vi "Get Ideal Aperture Time.vi"(0 "Measured Power (dBm)":dbl format="%#_13g", 5 "Total Aperture Time Limit (s)":dbl=120.0 format="%#_13g", 9 "Maximum Two Sigma Uncertainty (dB)":dbl=0.05 format="%#_13g", 11 "error in (no error)":errorcluster) -> (4 "Ideal Total Aperture time (s)":dbl, 6 "Ideal Number of Averages":dbl format="%.2f", 15 "error out":errorcluster)   [LabVIEW 2023, in "NI-568x RF Power Meter.lvlib" / "SG 2250 Path Accessor.lvclass"]
uses:
  SG 2250 Path Accessor.lvclass
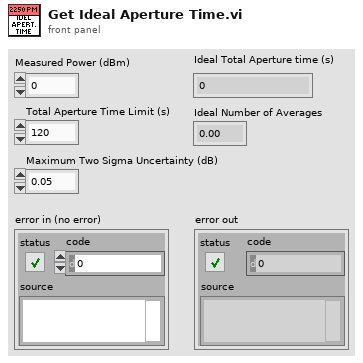
[diagram p1: front panel]
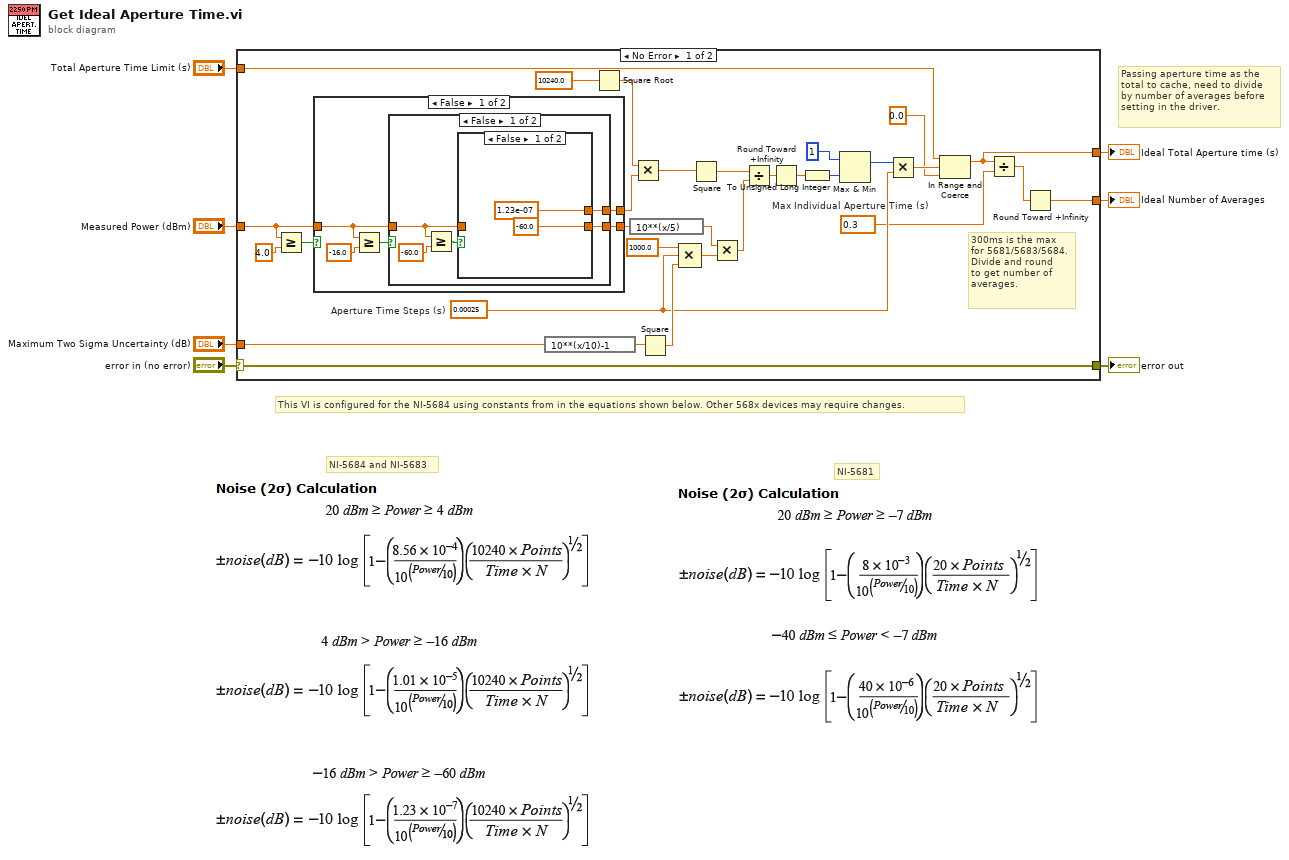
[diagram p0: block diagram]
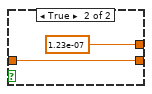
[diagram p2: hidden frame]
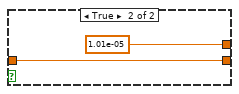
[diagram p3: hidden frame]
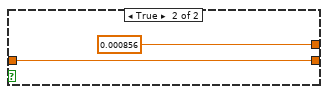
[diagram p4: hidden frame]
diagram:
  # "Passing aperture time as the\ntotal to cache, need to divide\nby number of averages before\nsetting in the driver."
  # "NI-5681"
  # "NI-5684 and NI-5683"
  # "This VI is configured for the NI-5684 using constants from in the equations shown below. Other 568x devices may require changes."
  n1 = case shown="No Error" "error in (no error)" {
    selector: "error in (no error)" -> [w16 w56]
    tunnel: "Measured Power (dBm)" -> [w32 _]
    tunnel: [w11 _] -> w6
    tunnel: [w16 w56] -> w4
    tunnel: [w13 _] -> w3
    tunnel: "Maximum Two Sigma Uncertainty (dB)" -> [w9 _]
    tunnel: "Total Aperture Time Limit (s)" -> [w8 _]
    frame No Error {
      w15 = 0.3  # Max Individual Aperture Time (s)
      w17 = 0.00025  # Aperture Time Steps (s)
      # "300ms is the max\nfor 5681/5683/5684.\nDivide and round\nto get number of\naverages."
      n2 = Greater Or Equal?(x=w32, y=4.0 ("upper limit")) -> (x >= y?=w34:bool)
      n3 = case shown="False" w34 {
        tunnel: w32 -> [w40 w55]
        tunnel: [w41 w55] -> w20
        tunnel: [w39 0.000856 ("t")] -> w33
        frame False {
          n4 = Greater Or Equal?(x=w40, y=-16.0 ("upper limit")) -> (x >= y?=w38:bool)
          n5 = case shown="False" w38 {
            tunnel: [w47 w52] -> w41
            tunnel: w40 -> [w44 w52]
            tunnel: [w46 1.01e-05 ("f")] -> w39
            frame False {
              n6 = Greater Or Equal?(x=w44, y=-60.0 ("upper limit")) -> (x >= y?=w43:bool)
              n7 = case shown="False" w43 {
                tunnel: [-60.0 ("Measured power (dBm)") w51] -> w47
                tunnel: [1.23e-07 ("f") 1.23e-07 ("f")] -> w46
                tunnel: w44 -> [_ w51]
                frame False {
                }
                frame True {
                }
              }
            }
            frame True {
            }
          }
        }
        frame True {
        }
      }
      n8 = expression code="10**(x/10)-1"(w9) -> (w26:dbl)
      n9 = Square Root(x=10240.0) -> (sqrt(x)=w35:dbl)
      n10 = expression code="10**(x/5)"(w20) -> (w29:dbl)
      n11 = Multiply(x=w35, y=w33) -> (x*y=w21:dbl)
      n12 = Square(x=w26) -> (x^2=w25:dbl)
      n13 = Compound Arithmetic op=MULTIPLY(1000.0 ("value"), w17, w25) -> (w19:dbl)
      n14 = Square(x=w21) -> (x^2=w27:dbl)
      n15 = Multiply(x=w29, y=w19) -> (x*y=w30:dbl)
      n16 = Divide(x=w27, y=w30) -> (x/y=w31:dbl)
      n17 = Round Toward +Infinity(x=w31) -> (ceil(x): smallest int >= x=w24:dbl)
      n18 = To Unsigned Long Integer(number=w24) -> (unsigned 32bit integer=w23:u32)
      n19 = Max & Min(x=u32 1, y=w23) -> (max(x,y)=w18:u32)  [unwired: 1 out]
      n20 = Multiply(x=w18, y=w17) -> (x*y=w12:dbl)
      n21 = In Range and Coerce(upper limit=w8, x=w12, lower limit=0.0) -> (coerced(x)=w11:dbl)  [unwired: 1 out]
      n22 = Divide(x=w11, y=w15) -> (x/y=w14:dbl)
      n23 = Round Toward +Infinity(x=w14) -> (ceil(x): smallest int >= x=w13:dbl)
    }
    frame Error {
    }
  }
  "Ideal Total Aperture time (s)" <- w6
  "error out" <- w4
  "Ideal Number of Averages" <- w3
